vi "CH_LM Config Data Header.vi"(0 "Meter Index":i32, 2 "Data Header (disable)":bool, 3 "Data Tokens":T1[](array[typedef]), 5 "error in (no error)":errorcluster, 7 "Timeout / ms (3000)":i32=3000, 8 "Action (query)":bool, 9 "Lock Timeout / ms (1000)":i32=1000) -> (11 "Lock timed out":bool, 14 "Meter Index":i32, 16 "Data Header":bool, 17 "Data Tokens":T1[](array[typedef]), 19 "error out":errorcluster)   [LabVIEW 2012, in "CH_LM.lvlib"]
doc: "This command will set/query whether data value identification strings will prefix data values reported over the host interface.\n\n<B>Note:</B> Headers will be in the form of \"<header>=<value>\". The <header> is literally one of the ID tag strings used in the data value send command.\n\n<B>Attention:</B> You should change data item selections only after ABORT and then only after flushing (reading) the remaining queued data. The next INIT will result in a data record format that you expect."
uses:
  CH_LM.lvlib
  _CH_LM/CH_LM Action Enumeration.ctl
  CH_LM Data Token.ctl
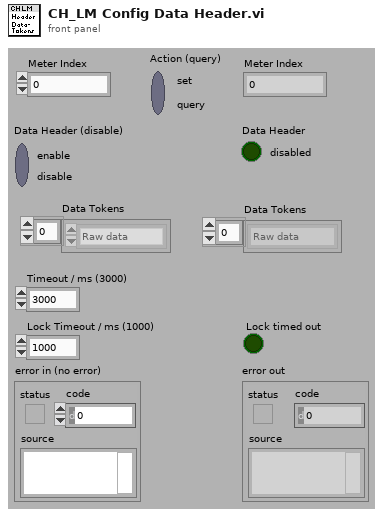
[diagram p1: front panel]
types:
  T1 = typedef "CH_LM.lvlib/CH_LM Data Token.ctl" = enum16{"Raw data", "Quad distance", "Formated data", "Unit", "Pulse period", "Flags", "Sequence ID"}
  T2 = typedef "CH_LM.lvlib/CH_LM Communication Mode.ctl" = enum16{"None", "USB", "GPIB", "RS232"}
  T3 = typedef "CH_LM.lvlib/CH_LM Action Enumeration.ctl" = enum16{"add", "read", "read by serial", "set", "remove", "delete", "Clear Shift-Register", ""}
  T4 = typedef "Semaphore RefNum" = refnum<k1>
  T5 = typedef "CH_LM.lvlib/CH_LM Meter Info.ctl" = cluster{"Meter Index":i32, "Serial Number":string, "Queue Cluster":T6, "Data Header":bool, "Data Tokens":T1[]}
  T6 = typedef "CH_LM.lvlib/CH_LM Queue Cluster.ctl" = cluster{"Streaming Queue":refnum<queue>, "Asynch Notifier":refnum<notifier>}
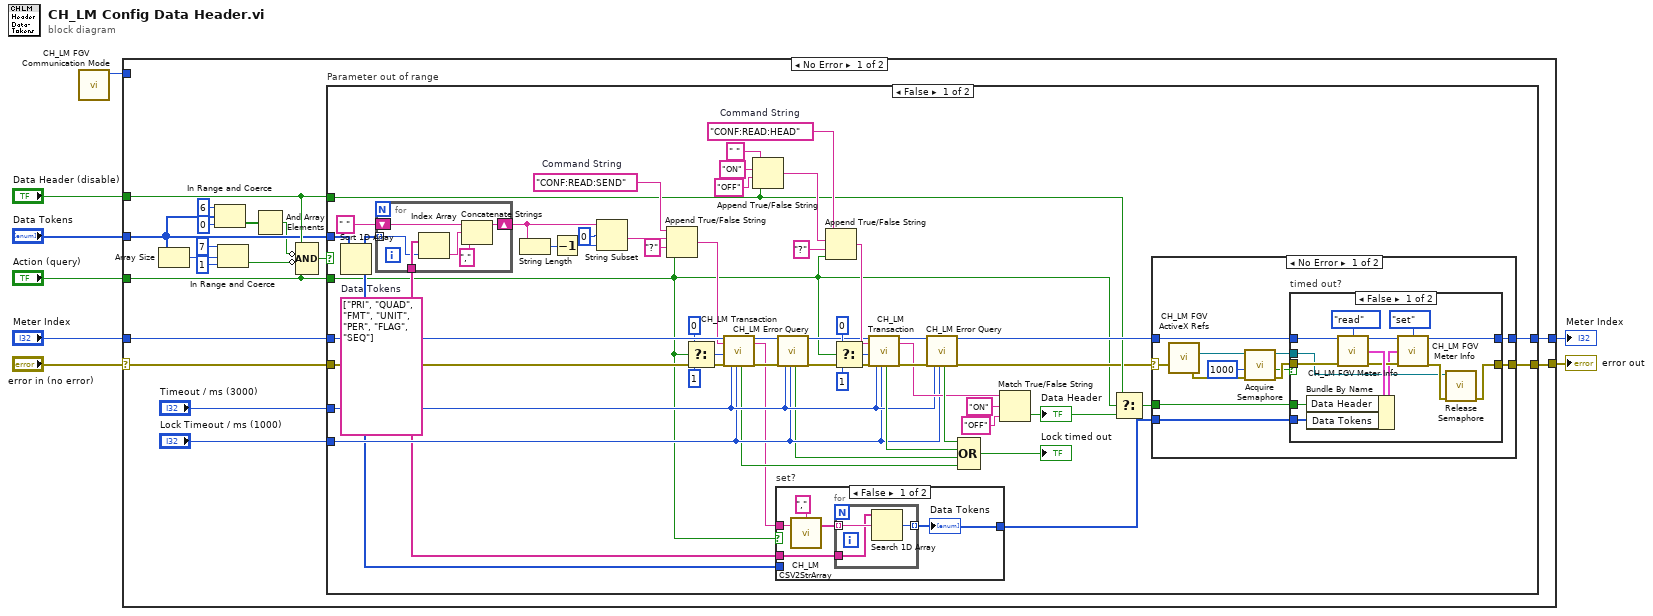
[diagram p0: block diagram]
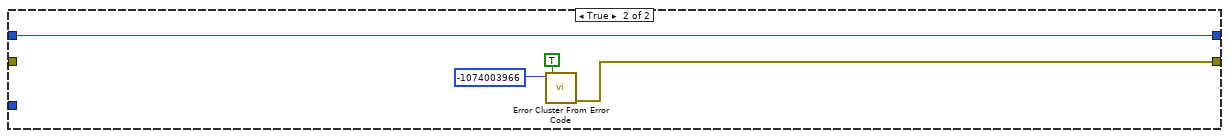
[diagram p5: hidden frame]
diagram:
  n1 = call "CH_LM FGV Communication Mode.vi"() -> ("Communication Mode"=w1:T2)  [unwired: 3 in, 5 out]
  n2 = case shown="No Error" "error in (no error)" {
    selector: "error in (no error)" -> [w26 w130]
    tunnel: [w24 w130] -> w8
    tunnel: "Meter Index" -> [w25 w129]
    tunnel: [w23 w129] -> w5
    tunnel: "Data Header (disable)" -> [w21 _]
    tunnel: "Action (query)" -> [w22 _]
    tunnel: "Data Tokens" -> [w20 _]
    tunnel: w1 -> [_ _]
    frame No Error {
      n3 = Array Size(array=w20) -> (size(s)=w18:i32)
      n4 = In Range and Coerce(upper limit=6, x=w20, lower limit=0) -> (In Range?=w9:bool[])  [unwired: 1 out]
      n5 = In Range and Coerce(upper limit=7, x=w18, lower limit=1) -> (In Range?=w17:bool)  [unwired: 1 out]
      n6 = And Array Elements(Boolean array=w9) -> (logical AND=w12:bool)
      n7 = Compound Arithmetic op=AND(w21, invert w12, invert w17, w22) -> (w19:bool)
      n8 = case "Parameter out of range" shown="False" w19 {
        tunnel: w26 -> [w60 _]
        tunnel: w25 -> [w61 w126]
        tunnel: [w30 w127] -> w24
        tunnel: [w29 w126] -> w23
        tunnel: w21 -> [w35 _]
        tunnel: w22 -> [w27 _]
        tunnel: w20 -> [w37 _]
        tunnel: "Timeout / ms (3000)" -> [w58 _]
        tunnel: "Lock Timeout / ms (1000)" -> [w57 _]
        frame False {
          w39 = string[] ["PRI", "QUAD", "FMT", "UNIT", "PER", "FLAG", "SEQ"]  # Data Tokens
          w43 = "CONF:READ:SEND"  # Command String
          w72 = "CONF:READ:HEAD"  # Command String
          n9 = Sort 1D Array(array=w37) -> (sorted array=w32:T1[])
          n10 = for {
            tunnel: w32 -> [w123] mode=indexing
            shift-right: [w122] -> w47
            shift-left: " " -> [w121]
            tunnel: w39 -> [w124]
            n11 = Index Array(array=w124, index=w123) -> (element=w120:string)
            n12 = Concatenate Strings(w121, w120, "," ("string")) -> (w122:string)
          }
          n13 = String Length(string=w47) -> (length=w48:i32)
          n14 = Decrement(x=w48) -> (x-1=w46:i32)
          n15 = String Subset(string=w47, offset (0)=0, length (rest)=w46) -> (substring=w42:string)
          n16 = Append True/False String(1:w27, 2:"?", 3:w42, 4:w43) -> (0:w41:string)
          n17 = Select(t=0, s=w27, f=1) -> (s? t:f=w53:i32)
          n18 = call "CH_LM Transaction.vi"("Meter Index"=w61, "Command String"=w41, "NofStrings (-1:all)"=w53, "error in (no error)"=w60, "Timeout / ms (3000)"=w58, "Lock Timeout / ms (1000)"=w57) -> ("Lock timed out"=w55:bool, "Meter Index"=w50:i32, "Response"=w40:string, "error out"=w51:errorcluster)  [unwired: 10 out]
          n19 = Append True/False String(1:w35, 2:"OFF" ("false string"), 3:"ON" ("true string"), 4:" " ("string (\"\")")) -> (0:w69:string)
          n20 = case "set?" shown="False" w27 {
            tunnel: w40 -> [w114 _]
            tunnel: w39 -> [w111 _]
            tunnel: w32 -> [_ w118]
            tunnel: [w110 w118] -> w31
            frame False {
              n21 = call "CH_LM CSV2StrArray.vi"("CSL"=w114, "Separator (,)"=",") -> ("Strings"=w112:string[])  [unwired: 1 in, 1 out]
              n22 = for {
                tunnel: w112 -> [w117] mode=indexing
                tunnel: w111 -> [w116]
                tunnel: [w115] -> w110 mode=indexing
                n23 = Search 1D Array(1D array=w116, element=w117) -> (index of element=w115:i32)  [unwired: 1 out]
              }
              "Data Tokens" <- w110
            }
            frame True {
            }
          }
          n24 = call "CH_LM Error Query.vi"("Meter Index"=w50, "error in (no error)"=w51, "Timeout / ms (3000)"=w58, "Lock Timeout / ms (1000)"=w57) -> ("Lock timed out"=w56:bool, "Meter Index"=w59:i32, "error out"=w38:errorcluster)  [unwired: 13 out]
          n25 = Append True/False String(1:w27, 2:"?", 3:w69, 4:w72) -> (0:w68:string)
          n26 = Select(t=0, s=w27, f=1) -> (s? t:f=w66:i32)
          n27 = call "CH_LM Transaction.vi"("Meter Index"=w59, "Command String"=w68, "NofStrings (-1:all)"=w66, "error in (no error)"=w38, "Timeout / ms (3000)"=w58, "Lock Timeout / ms (1000)"=w57) -> ("Lock timed out"=w76:bool, "Meter Index"=w79:i32, "Response"=w64:string, "error out"=w78:errorcluster)  [unwired: 10 out]
          n28 = call "CH_LM Error Query.vi"("Meter Index"=w79, "error in (no error)"=w78, "Timeout / ms (3000)"=w58, "Lock Timeout / ms (1000)"=w57) -> ("Lock timed out"=w77:bool, "Meter Index"=w36:i32, "error out"=w28:errorcluster)  [unwired: 13 out]
          n29 = Compound Arithmetic op=OR(w77, w76, w56, w55) -> (→"Lock timed out":bool)
          n30 = Match True/False String(2:"OFF" ("false string"), 3:"ON" ("true string"), 4:w64) -> (0:w34:bool)  [unwired: 1 out]
          "Data Header" <- w34
          n31 = Select(t=w35, s=w27, f=w34) -> (s? t:f=w33:bool)
          n32 = case shown="No Error" w28 {
            selector: w28 -> [w80 w108]
            tunnel: w36 -> [w88 w109]
            tunnel: w33 -> [w86 _]
            tunnel: w31 -> [w85 _]
            tunnel: [w84 w108] -> w30
            tunnel: [w82 w109] -> w29
            frame No Error {
              n33 = call "CH_LM FGV ActiveX Refs.vi"("error in (no error)"=w80) -> ("error out"=w90:errorcluster, "CH_LM semaphore"=w91:T4)  [unwired: 4 in, 2 out]
              n34 = call <vilib>:"Acquire Semaphore.vi"("error in (no error)"=w90, "ms timeout (-1)"=1000, "semaphore"=w91) -> ("error out"=w87:errorcluster, "timed out"=w83:bool, "semaphore out"=w81:T4)  [unwired: 2 out]
              n35 = case "timed out?" shown="False" w83 {
                tunnel: w88 -> [w105 w106]
                tunnel: w87 -> [w104 w107]
                tunnel: w86 -> [w101 _]
                tunnel: w85 -> [w100 _]
                tunnel: [w93 w107] -> w84
                tunnel: [w95 w106] -> w82
                tunnel: w81 -> [w92 _]
                frame False {
                  n36 = call "CH_LM FGV Meter Info.vi"("Meter Index"=w105, "Action (read)"=CH_LM_Action_Enumeration."read", "error in (no error)"=w104) -> ("Meter Index out"=w99:i32, "Meter Info"=w102:T5, "error out"=w98:errorcluster)  [unwired: 2 in, 8 out]
                  n37 = Bundle By Name(cluster=w102, "Data Header"=w101, "Data Tokens"=w100) -> (w97:T5)
                  n38 = call "CH_LM FGV Meter Info.vi"("Meter Index"=w99, "Action (read)"=CH_LM_Action_Enumeration."set", "Meter Info"=w97, "error in (no error)"=w98) -> ("Meter Index out"=w95:i32, "error out"=w94:errorcluster)  [unwired: 1 in, 9 out]
                  n39 = call <vilib>:"Release Semaphore.vi"("error in (no error)"=w94, "semaphore"=w92) -> ("error out"=w93:errorcluster)  [unwired: 5 out]
                }
                frame True {
                }
              }
            }
            frame Error {
            }
          }
        }
        frame True {
          n40 = call <vilib>:"Error Cluster From Error Code.vi"("show call chain? (False)"=TRUE, "error code (0)"=-1074003966) -> ("error out"=w127:errorcluster)  [unwired: 1 in, 6 out]
        }
      }
    }
    frame Error {
    }
  }
  "error out" <- w8
  "Meter Index" <- w5
